vi "test-linear-filter-test-03-funcA.vi"(11 "Input":dbl) -> (3 "Output":dbl)   [LabVIEW 2019]
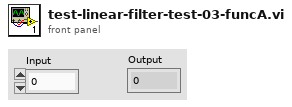
[diagram p1: front panel]
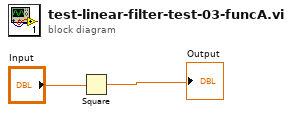
[diagram p0: block diagram]
diagram:
  n1 = Square(x="Input") -> (x^2=→"Output":dbl)
